vi "Handle Command.vi"(8 "error in (no error)":errorcluster, 9 "Data":variant, 10 "Command":string, 11 "VoltageUpdate":refnum<class "VoltageUpdate.lvclass">) -> (0 "error out":errorcluster, 1 "Processed Data":variant, 2 "Command":string, 3 "VoltageUpdate out":refnum<class "VoltageUpdate.lvclass">)   [LabVIEW 2016, in "VoltageUpdate.lvclass"]
uses:
  VoltageUpdate.lvclass
  VoltageUpdate.lvclass/VoltageUpdate.ctl
  <userlib>/LevyLab/Levylab Instruments/Instrument Types/VSource/Instrument.VSource.lvclass
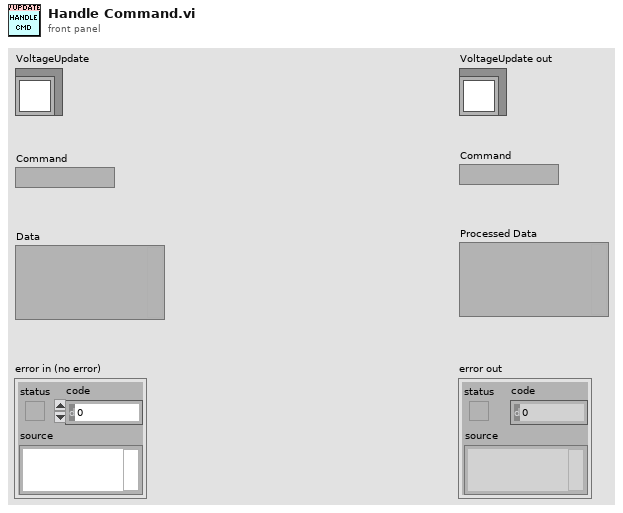
[diagram p1: front panel]
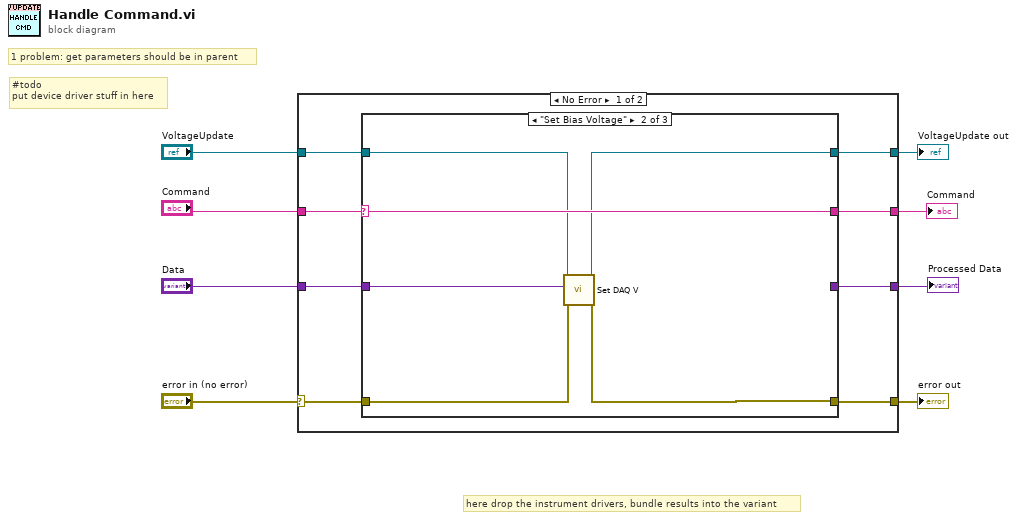
[diagram p0: block diagram]
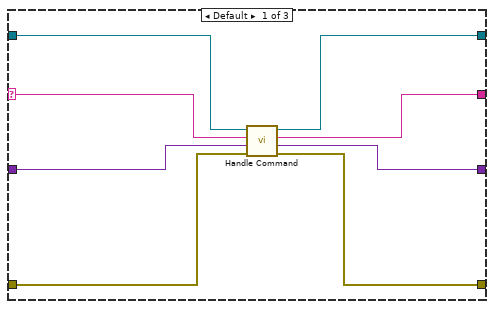
[diagram p2: hidden frame]
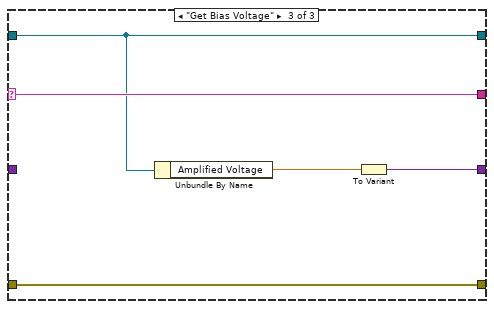
[diagram p3: hidden frame]
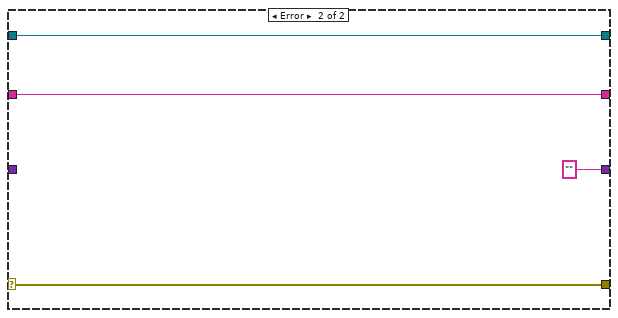
[diagram p4: hidden frame]
diagram:
  # "here drop the instrument drivers, bundle results into the variant"
  # "1 problem: get parameters should be in parent"
  # "#todo\nput device driver stuff in here"
  n1 = case shown="No Error" "error in (no error)" {
    selector: "error in (no error)" -> [w12 w39]
    tunnel: [w10 w39] -> w6
    tunnel: [w14 w38] -> w5
    tunnel: "VoltageUpdate" -> [w15 w38]
    tunnel: "Command" -> [w16 w36]
    tunnel: [w13 "" ("String")] -> w3
    tunnel: "Data" -> [w11 _]
    tunnel: [w9 w36] -> w1
    frame No Error {
      n2 = case shown="\"Set Bias Voltage\"" w16 {
        selector: w16 -> [w24 w30 w34]
        tunnel: w15 -> [w21 w28 w33]
        tunnel: [w18 w27 w33] -> w14
        tunnel: [w20 _ w31] -> w13
        tunnel: w12 -> [w22 w29 w35]
        tunnel: w11 -> [w23 w25 _]
        tunnel: [w19 w26 w35] -> w10
        tunnel: [w17 w30 w34] -> w9
        frame Default {
          n3 = call-parent "Handle Command.vi"("error in (no error)"=w22, "Data"=w23, "Command"=w24, "Instrument in"=w21) -> ("error out"=w19:errorcluster, "Processed Data"=w20:variant, "Command"=w17:string, "Instrument out"=w18:refnum<class "VoltageUpdate.lvclass">)  [unwired: 4 in]
        }
        frame "Set Bias Voltage" {
          n4 = call "Set DAQ V.vi"("error in (no error)"=w29, "Set Voltage"=w25, "VoltageUpdate in"=w28) -> ("error out"=w26:errorcluster, "VoltageUpdate out"=w27:refnum<class "VoltageUpdate.lvclass">)  [unwired: 7 in]
        }
        frame "Get Bias Voltage" {
          n5 = Unbundle By Name(w33) -> ("Amplified Voltage"=w32:dbl)
          n6 = To Variant(anything=w32) -> (Variant=w31:variant)
        }
      }
    }
    frame Error {
    }
  }
  "error out" <- w6
  "VoltageUpdate out" <- w5
  "Command" <- w1
  "Processed Data" <- w3
